vi "Set Exposure Time.vi"(8 "Error in":errorcluster, 10 "Exposure Time":dbl[unit]=1.0, 11 "Com in":refnum<visa-resource-name>) -> (0 "Error out":errorcluster, 3 "Com out":refnum<visa-resource-name>)   [LabVIEW 2020]
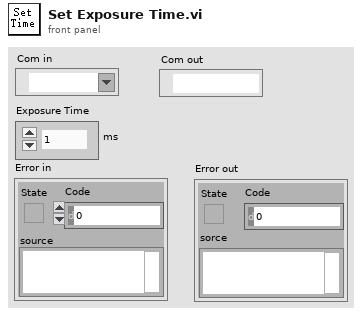
[diagram p1: front panel]
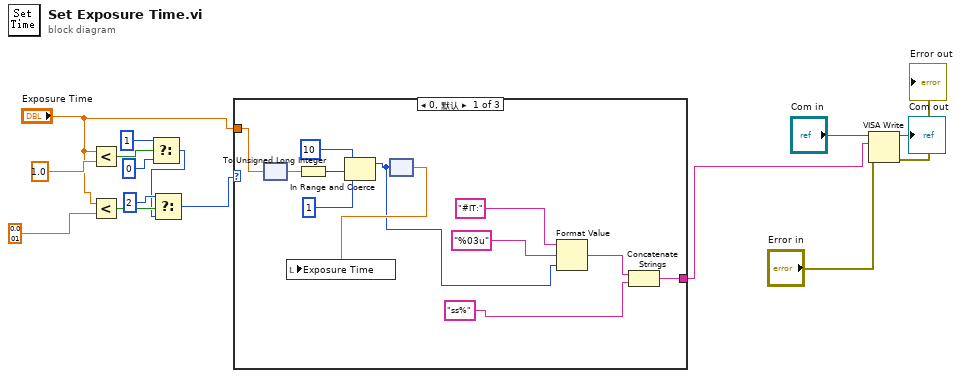
[diagram p0: block diagram]
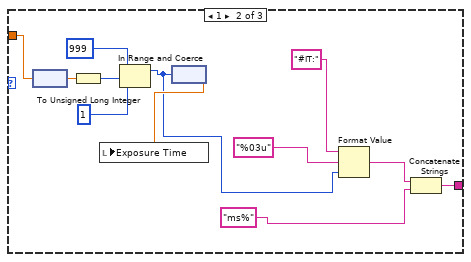
[diagram p2: hidden frame]
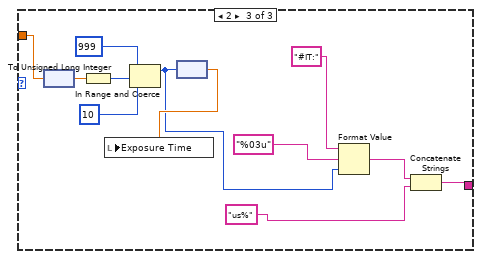
[diagram p3: hidden frame]
diagram:
  n1 = Less?(x="Exposure Time", y=dbl[unit] 1.0) -> (x < y?=w10:bool)
  n2 = Less?(x="Exposure Time", y=dbl[unit] 0.001) -> (x < y?=w7:bool)
  n3 = Select(t=1, s=w10, f=0) -> (s? t:f=w4:i32)
  n4 = Select(t=2 ("f"), s=w7, f=w4) -> (s? t:f=w3:i32)
  n5 = case shown="0, 默认" w3 {
    tunnel: "Exposure Time" -> [w27 w39 w51]
    tunnel: [w17 w30 w41] -> w1
    frame 0, Default {
      n6 = node(w27) -> (w26:dbl)
      n7 = To Unsigned Long Integer(number=w26) -> (unsigned 32bit integer=w25:u32)
      n8 = In Range and Coerce(upper limit=u32 10 ("上限"), x=w25, lower limit=u32 1 ("下限")) -> (coerced(x)=w16:u32)  [unwired: 1 out]
      n9 = node(w16) -> (w22:dbl[unit])
      n10 = local write "Exposure Time"(w22) -> ()
      n11 = Format Value(string ("")="#IT:" ("字符串(\"\")"), format string="%03u" ("格式字符串"), value (0)=w16) -> (output string=w18:string)
      n12 = Concatenate Strings(w18, "ss%" ("字符串")) -> (w17:string)
    }
    frame 1 {
      n13 = node(w39) -> (w38:dbl)
      n14 = To Unsigned Long Integer(number=w38) -> (unsigned 32bit integer=w37:u32)
      n15 = In Range and Coerce(upper limit=u32 999 ("上限"), x=w37, lower limit=u32 1 ("下限")) -> (coerced(x)=w29:u32)  [unwired: 1 out]
      n16 = node(w29) -> (w34:dbl[unit])
      n17 = local write "Exposure Time"(w34) -> ()
      n18 = Format Value(string ("")="#IT:" ("字符串(\"\")"), format string="%03u" ("格式字符串"), value (0)=w29) -> (output string=w33:string)
      n19 = Concatenate Strings(w33, "ms%" ("字符串")) -> (w30:string)
    }
    frame 2 {
      n20 = node(w51) -> (w50:dbl)
      n21 = To Unsigned Long Integer(number=w50) -> (unsigned 32bit integer=w49:u32)
      n22 = In Range and Coerce(upper limit=u32 999 ("上限"), x=w49, lower limit=u32 10 ("下限")) -> (coerced(x)=w40:u32)  [unwired: 1 out]
      n23 = node(w40) -> (w46:dbl[unit])
      n24 = local write "Exposure Time"(w46) -> ()
      n25 = Format Value(string ("")="#IT:" ("字符串(\"\")"), format string="%03u" ("格式字符串"), value (0)=w40) -> (output string=w42:string)
      n26 = Concatenate Strings(w42, "us%" ("字符串")) -> (w41:string)
    }
  }
  n27 = VISA Write(VISA resource name="Com in", write buffer=w1, error in (no error)="Error in") -> (VISA resource name out=→"Com out":refnum<visa-resource-name>, error out=→"Error out":errorcluster)  [unwired: 1 out]
